vi "HandleItemActivation.vi"(8 "error in (no error)":errorcluster, 11 "Error in":refnum<class "Error.lvclass">) -> (0 "error out":errorcluster, 3 "Error out":refnum<class "Error.lvclass">)   [LabVIEW 2009, in "NavScreen.lvlib" / "Error.lvclass"]
uses:
  Error.lvclass
  Error.lvclass/Error.ctl
panel:
  in  "Message":string="The Handler \"%s\" is not correctly defined in the XML file. Alternatively, if this is a valid handler, it may not be associated with a LabVIEW Class object in %s."
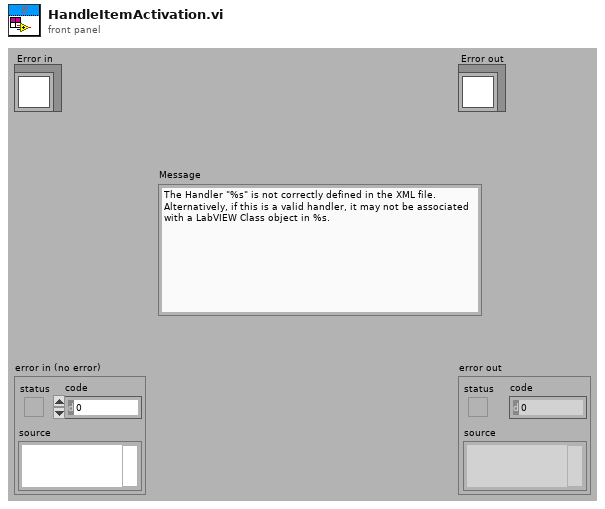
[diagram p1: front panel]
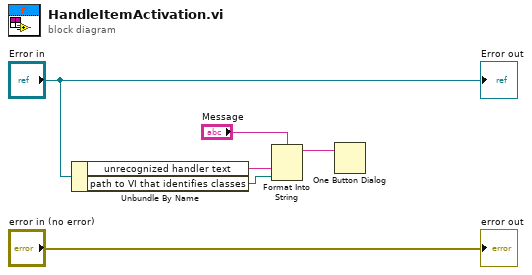
[diagram p0: block diagram]
diagram:
  n1 = Unbundle By Name("Error in") -> ("unrecognized handler text"=w4:string, "path to VI that identifies classes"=w3:path)
  n2 = Format Into String(format string="Message", w4, w3) -> (resulting string=w2:string)  [unwired: 2 in, 1 out]
  n3 = One Button Dialog(message=w2) -> ()  [unwired: 1 in, 1 out]
  "error out" <- "error in (no error)"
  "Error out" <- "Error in"
